vi "removeEdge.vi"(0 "reference":refnum<class "Graph.lvclass">, 1 "edge":refnum<class "AbstractEdge.lvclass">, 5 "error in (no error)":errorcluster) -> (14 "reference out":refnum<class "Graph.lvclass">, 19 "error out":errorcluster)   [LabVIEW 2016, in "Graph.lvclass"]
doc: "public void removeEdge(Edge e)"
uses:
  <resource>/Framework/Providers/Open_GDS/UML/Graph_class/Graph.lvclass
  <resource>/Framework/Providers/Open_GDS/UML/AbstractEdge_class/AbstractEdge.lvclass
  <resource>/Framework/Providers/Open_GDS/UML/AbstractNode_class/AbstractNode.lvclass
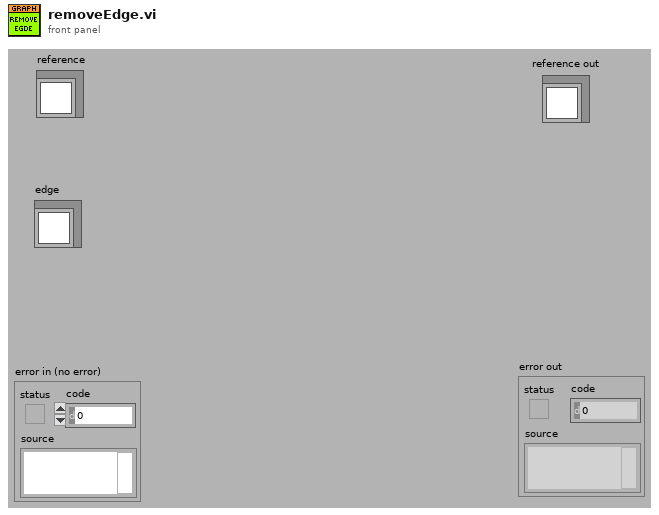
[diagram p1: front panel]
types:
  T1 = typedef "Graph.lvclass/ObjectAttributes.ctl" = cluster{"nodes":refnum<class "AbstractNode.lvclass">[], "edges":refnum<class "AbstractEdge.lvclass">[], "nodesToBeRemoved":refnum<class "AbstractNode.lvclass">[], "edgesToBeRemoved":refnum<class "AbstractEdge.lvclass">[], "needsLayout":bool, "LayoutNodes":refnum<class "AbstractNode.lvclass">[]}
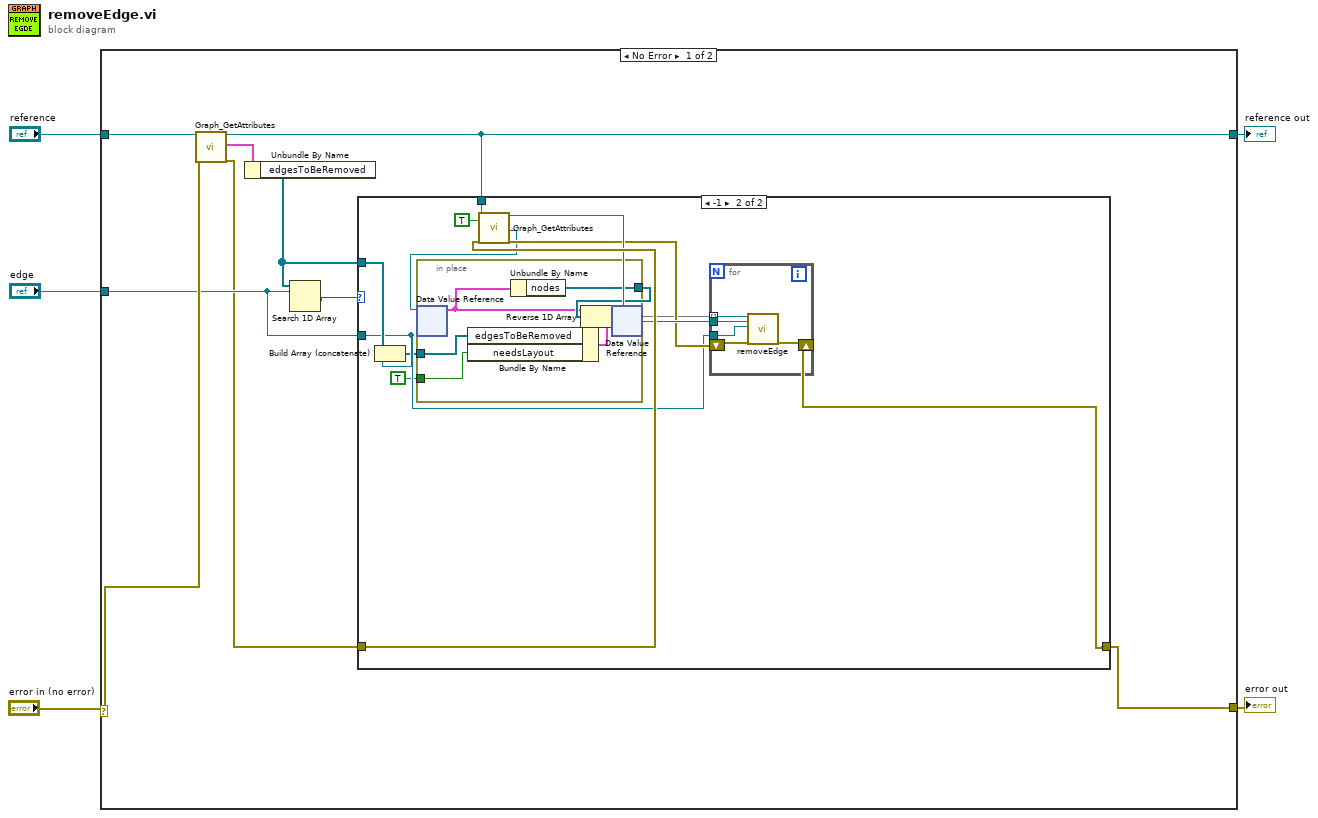
[diagram p0: block diagram]
diagram:
  n1 = case shown="No Error" "error in (no error)" {
    selector: "error in (no error)" -> [w11 w39]
    tunnel: "reference" -> [w14 w40]
    tunnel: [w13 w39] -> w4
    tunnel: [w12 w40] -> w3
    tunnel: "edge" -> [w10 _]
    frame No Error {
      n2 = call <resource>:"Graph_GetAttributes.vi"("reference in"=w14, "error in (no error)"=w11) -> ("reference out"=w12:refnum<class "Graph.lvclass">, "Data"=w6:T1, "error out"=w8:errorcluster)  [unwired: 1 in, 14 out]
      n3 = Unbundle By Name(w6) -> ("edgesToBeRemoved"=w7:refnum<class "AbstractEdge.lvclass">[])
      n4 = Search 1D Array(1D array=w7, element=w10) -> (index of element=w9:i32)  [unwired: 1 out]
      n5 = case shown="-1" w9 {
        tunnel: w8 -> [w15 w27]
        tunnel: [w15 w21] -> w13
        tunnel: w12 -> [_ w28]
        tunnel: w7 -> [_ w26]
        tunnel: w10 -> [_ w23]
        frame 0, Default {
        }
        frame -1 {
          n6 = Build Array (concatenate)(w26, w23) -> (w17:refnum<class "AbstractEdge.lvclass">[])
          n7 = call <resource>:"Graph_GetAttributes.vi"("reference in"=w28, "OnlyGetDvrReference(False)"=TRUE, "error in (no error)"=w27) -> ("reference out"=w25:refnum<class "Graph.lvclass">, "DataRef"=w19:refnum<data-value>, "error out"=w24:errorcluster)  [unwired: 13 in, 1 out]
          n8 = in-place {
            in-place-border: [w32] -> w18
            in-place-border: w17 -> [w31]
            in-place-border: TRUE ("needsLayout") -> [w30]
            n9 = in-place-dvr #1(w19) -> (w33:T1)  [unwired: 1 out]
            n10 = Bundle By Name(cluster=w33, "edgesToBeRemoved"=w31, "needsLayout"=w30) -> (w29:T1)
            n11 = Unbundle By Name(w33) -> ("nodes"=w32:refnum<class "AbstractNode.lvclass">[])
            n12 = in-place-dvr #1(w29) -> ()  [unwired: 2 out]
          }
          n13 = Reverse 1D Array(array=w18) -> (reversed array=w22:refnum<class "AbstractNode.lvclass">[])
          n14 = for {
            tunnel: w22 -> [w38] mode=indexing
            tunnel: w25 -> [w37]
            tunnel: w23 -> [w36]
            shift-right: [w34] -> w21
            shift-left: w24 -> [w35]
            n15 = call-dynamic "removeEdge.vi"("reference"=w38, "graph"=w37, "edge"=w36, "error in (no error)"=w35) -> ("error out"=w34:errorcluster)  [unwired: 14 in, 1 out]
          }
        }
      }
    }
    frame Error {
    }
  }
  "reference out" <- w3
  "error out" <- w4
